vi "add new channel.vi"(8 "error in":errorcluster, 10 "TBM channel in":refnum<class "TBM channel.lvclass">, 11 "TDMS datalogger editor node in":refnum<class "TDMS datalogger editor node.lvclass">) -> (0 "error out":errorcluster, 3 "TDMS datalogger editor node out":refnum<class "TDMS datalogger editor node.lvclass">)   [LabVIEW 2013]
uses:
  TDMS datalogger editor node.lvclass
  <vilib>/NI/TBM Modules/TDMS Datalogger/module/configuration/TDMS datalogger configuration.lvclass
  <vilib>/NI/Tag Bus Module Framework/channel/TBM channel.lvclass
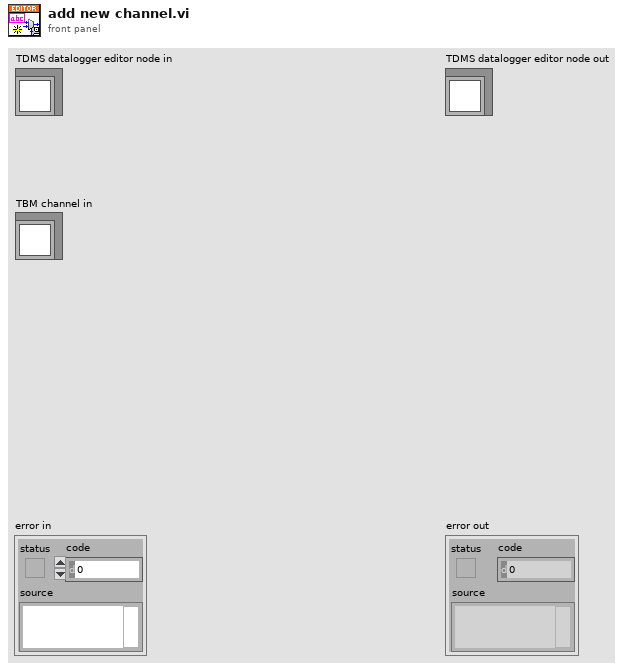
[diagram p1: front panel]
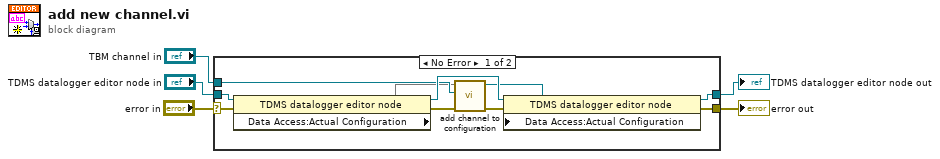
[diagram p0: block diagram]
diagram:
  n1 = case shown="No Error" "error in" {
    selector: "error in" -> [w15 w16]
    tunnel: "TDMS datalogger editor node in" -> [w11 w17]
    tunnel: [w13 w17] -> w3
    tunnel: [w14 w16] -> w2
    tunnel: "TBM channel in" -> [w10 _]
    frame No Error {
      n2 = property class="TDMS datalogger editor node"(reference=w11, error in=w15) -> (reference out=w12:refnum<class "TDMS datalogger editor node.lvclass">, error out=w6:errorcluster, "Data Access:Actual Configuration"=w9)
      n3 = call <vilib>:"add channel to configuration.vi"("error in"=w6, "TBM channel in"=w10, "TDMS datalogger configuration in"=w9) -> ("error out"=w7:errorcluster, "TDMS datalogger configuration out"=w8:refnum<class "TDMS datalogger configuration.lvclass">)  [unwired: 7 in]
      n4 = property class="TDMS datalogger editor node"(reference=w12, error in=w7, "Data Access:Actual Configuration"=w8) -> (reference out=w13:refnum<class "TDMS datalogger editor node.lvclass">, error out=w14:errorcluster)
    }
    frame Error {
    }
  }
  "error out" <- w2
  "TDMS datalogger editor node out" <- w3
